vi "Rotate CW.vi"(10 "Direction":T1) -> (2 "CW Rotated":T1)   [LabVIEW 2020, in "SquareBattle.lvlib"]
doc: "Returns the direction that is 45 degrees clockwise from the specified direction. E.g. if N is specified, NE will be returned and if W is specified NW will be returned."
uses:
  SquareBattle.lvlib
  Direction.ctl
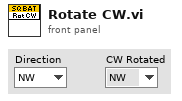
[diagram p1: front panel]
types:
  T1 = typedef "SquareBattle.lvlib/Direction.ctl" = enum16{"NW", "N", "NE", "E", "SE", "S", "SW", "W"}
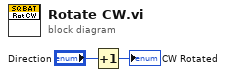
[diagram p0: block diagram]
diagram:
  n1 = Increment(x="Direction") -> (x+1=→"CW Rotated":T1)
